vi "Render.vi"(0 "class data in":refnum<class "SceneRoot.lvclass">, 5 "error in (no error)":errorcluster) -> (14 "class data out":refnum<class "SceneRoot.lvclass">, 19 "error out":errorcluster)   [LabVIEW 2010, in "RenderBase.lvlib" / "SceneRoot.lvclass"]
doc: "Renders the scene."
uses:
  SceneRoot.lvclass
  SceneRoot.lvclass/SceneRoot.ctl
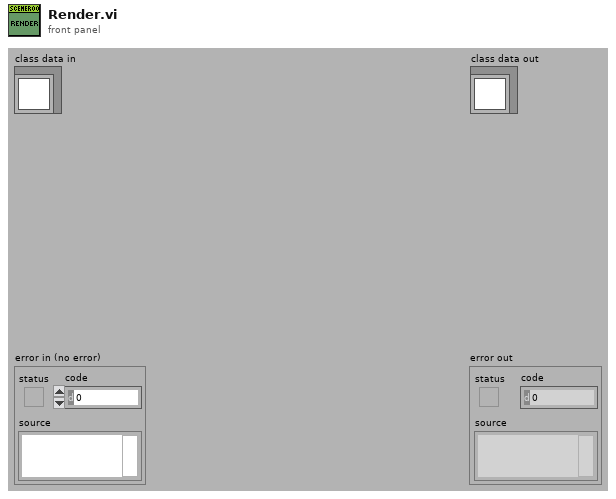
[diagram p1: front panel]
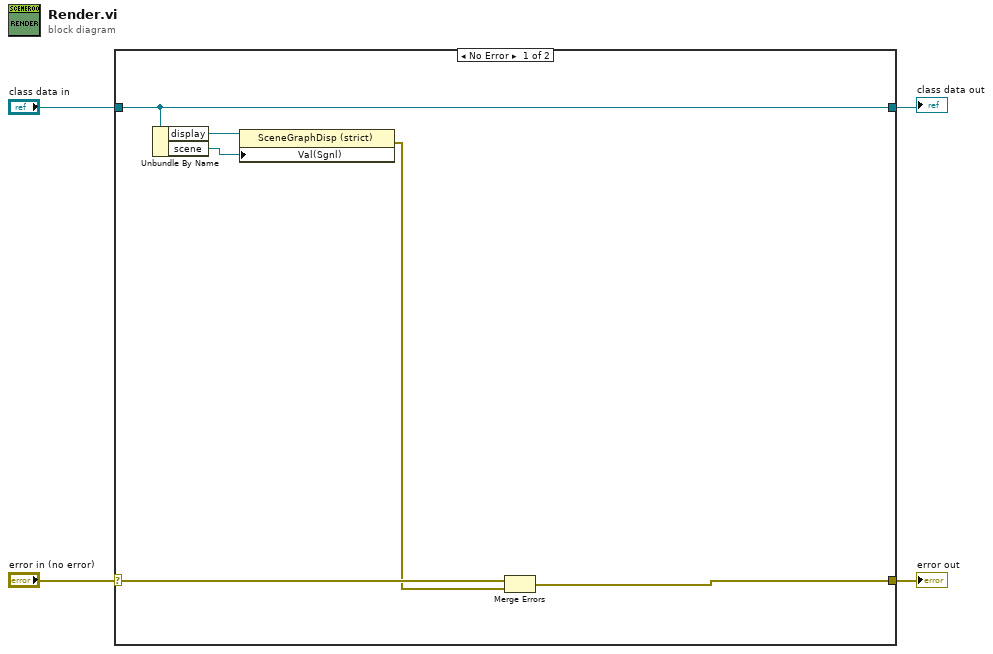
[diagram p0: block diagram]
diagram:
  n1 = case shown="No Error" "error in (no error)" {
    selector: "error in (no error)" -> [w10 w12]
    tunnel: [w6 w12] -> w3
    tunnel: "class data in" -> [w9 w11]
    tunnel: [w9 w11] -> w1
    frame No Error {
      n2 = Unbundle By Name(w9) -> ("display"=w8:refnum<vi>, "scene"=w7:refnum<vi>)
      n3 = property class="SceneGraphDisp (strict)"(reference=w8, "Val(Sgnl)"=w7) -> (error out=w5:errorcluster)  [unwired: 1 in, 1 out]
      n4 = Merge Errors(w10, w5) -> (w6:errorcluster)
    }
    frame Error {
    }
  }
  "error out" <- w3
  "class data out" <- w1
